vi "Turn To Vision.vi"() -> (1 "Motor Powers":cluster{"Left Motor":dbl, "Right Motor":dbl}, 3 "Done":bool)   [LabVIEW 2016]
uses:
  Vision Global.vi
  <vilib>/addons/control/pid/pid.llb/PID (DBL).vi
  <vilib>/addons/control/pid/NI_PID_pid.lvlib
  <vilib>/ptbypt/NI_PtbyPt.lvlib
panel:
  in  "Time Target (s)":dbl=0.15 format="%#_13g"
  out "Elapsed Time (s)":dbl
  in  "PID gains":T1={"proportional gain (Kc)"=1.0, "integral time (Ti, min)"=0.01, "derivative time (Td, min)"=0.0} {"derivative time (Td, min)" format="%.3f"; "integral time (Ti, min)" format="%.3f"; "proportional gain (Kc)" format="%.3f"}
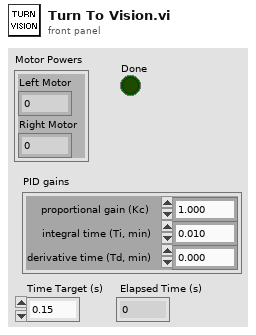
[diagram p1: front panel]
types:
  T1 = cluster{"proportional gain (Kc)":dbl, "integral time (Ti, min)":dbl, "derivative time (Td, min)":dbl}
  T2 = cluster{"Distance (ft)":dbl, "Score":dbl, "Normalized":cluster{"Center":cluster{dbl, dbl}, "Rectangle":cluster{"Numeric":dbl, "Numeric 2":dbl, "Numeric 3":dbl, "Numeric 5":dbl}}, "Pixels":cluster{"Center":cluster{dbl, dbl}, "Rectangle":cluster{"Numeric":dbl, "Numeric 2":dbl, "Numeric 3":dbl, "Numeric 5":dbl}}}
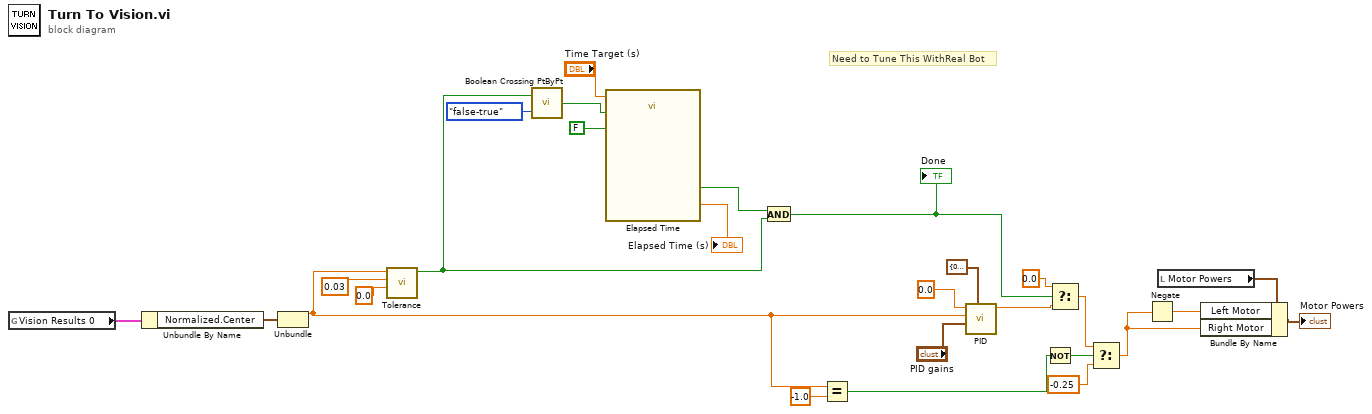
[diagram p0: block diagram]
diagram:
  # "Need to Tune This WithReal Bot"
  n1 = global read "Vision Global.vi" "Vision Results 0"() -> (w27:T2)
  n2 = Unbundle By Name(w27) -> ("Normalized.Center"=w26:cluster{dbl, dbl})
  n3 = Unbundle(w26) -> (w7:dbl)  [unwired: 1 out]
  n4 = call "Tolerance.vi"("Setpoint"=0.0, "Tolerance"=0.03, "Current Value"=w7) -> ("In Range?"=w20:bool)  [unwired: 8 in]
  n5 = call <vilib>:"Boolean Crossing PtByPt.vi"("direction"=enum16{"either", "false-true", "true-false"}."false-true", "input"=w20) -> ("crossing"=w18:bool)  [unwired: 1 in]
  n6 = call "Elapsed Time"("Time Target (s)"="Time Target (s)", "Reset"=w18, "Auto Reset"=FALSE) -> ("Elapsed Time (s)"=→"Elapsed Time (s)":dbl, "Time has Elapsed"=w15:bool)  [unwired: 9 in, 6 out]
  n7 = And(x=w15, y=w20) -> (x .and. y?=w11:bool)
  "Done" <- w11
  n8 = Equal?(x=w7, y=-1.0) -> (x = y?=w5:bool)
  n9 = call-poly <vilib>:"PID.vi"("output range"=cluster{"output high":dbl, "output low":dbl} {"output high"=0.8, "output low"=-0.8}, "PID gains"="PID gains", "process variable"=w7, "setpoint"=0.0) -> ("output"=w12:dbl)  [unwired: 6 in, 1 out]
  n10 = Not(x=w5) -> (.not. x?=w3:bool)
  n11 = Select(t=0.0, s=w11, f=w12) -> (s? t:f=w4:dbl)
  n12 = Select(t=w4, s=w3, f=-0.25) -> (s? t:f=w1:dbl)
  n13 = Negate(x=w1) -> (-x=w8:dbl)
  n14 = local read "Motor Powers"() -> (w23:cluster{"Left Motor":dbl, "Right Motor":dbl})
  n15 = Bundle By Name(cluster=w23, "Left Motor"=w8, "Right Motor"=w1) -> (→"Motor Powers":cluster{"Left Motor":dbl, "Right Motor":dbl})
